vi "Write test data to sql database.vi"(6 "error in (no error)":errorcluster, 9 "Serial":string) -> (0 "error out":errorcluster, 1 "No dup serial?":bool, 2 "Test rec csv line":string, 3 "Passed?":bool)   [LabVIEW 2013]
uses:
  Test Globals/Global 1.vi
  Main Support/Global 2.vi
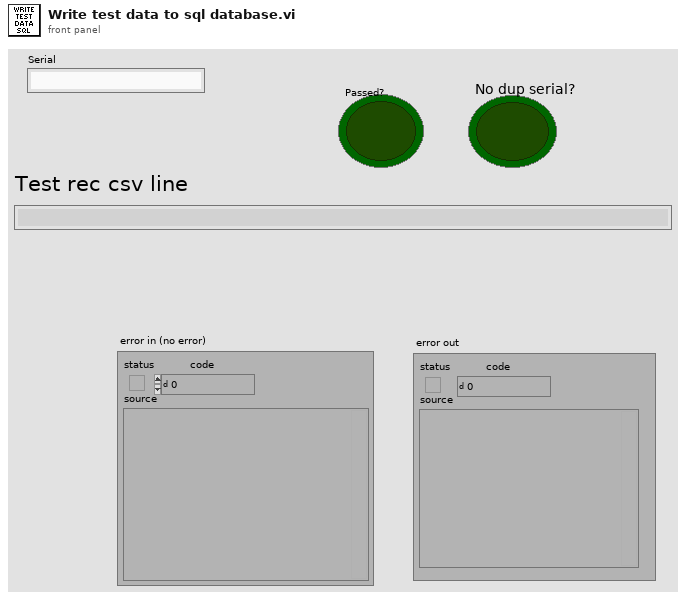
[diagram p1: front panel]
types:
  T1 = enum16{"Query", "Insert", "Select", "Dump Recs", "Get Rec Count", "Get Col Names", "Insert all fields", "Find", "Get last test result", "Get work order qty", "Set work order qty", "Save test report", "Get test report", "Execute query no data", "Select count", "Query and return row 0 col 0"}
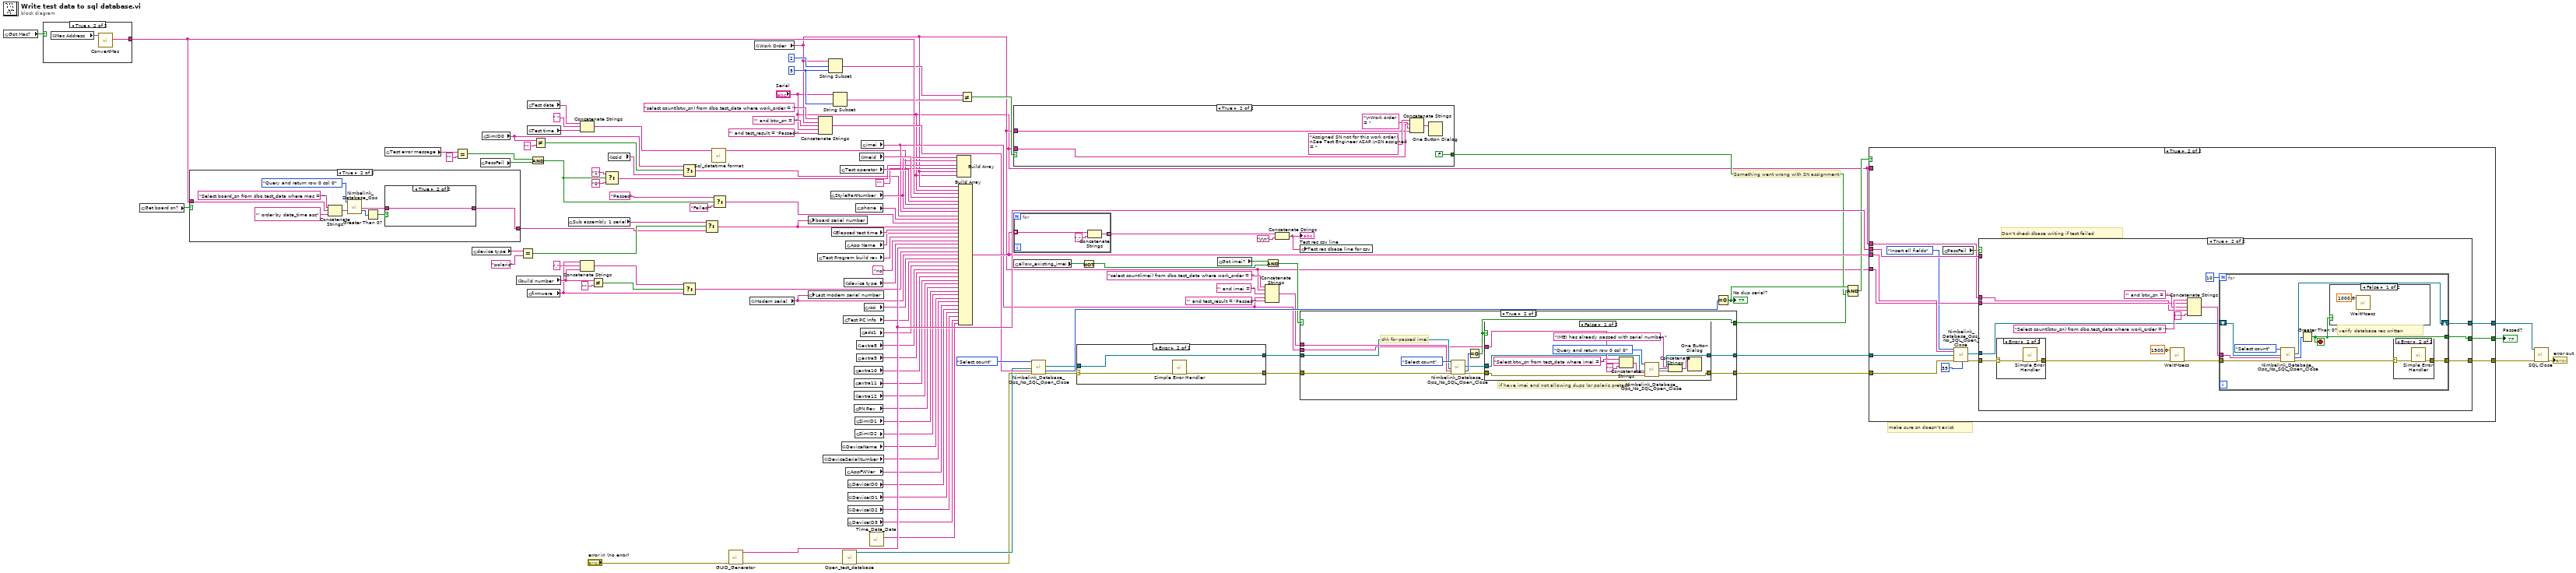
[diagram p0: block diagram]
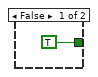
[diagram p2: hidden frame]
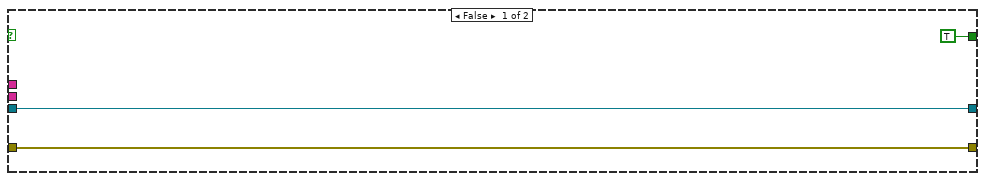
[diagram p3: hidden frame]
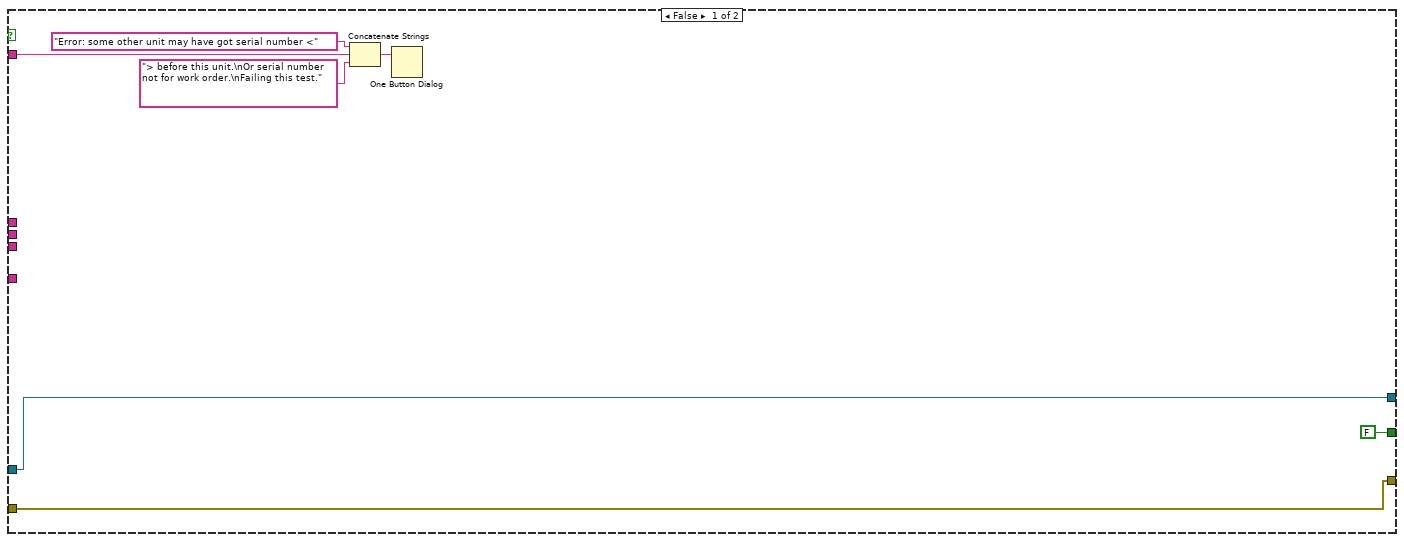
[diagram p6: hidden frame]
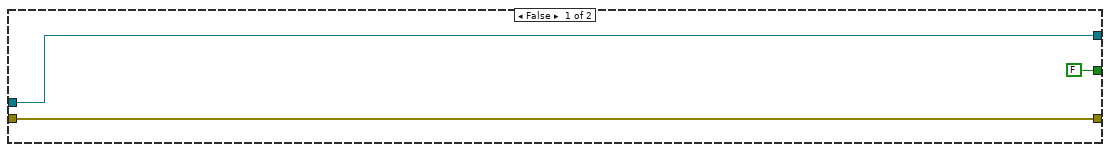
[diagram p7: hidden frame]
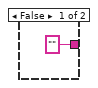
[diagram p11: hidden frame]
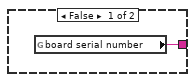
[diagram p12: hidden frame]
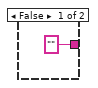
[diagram p13: hidden frame]
diagram:
  w55 = 5 ("length (rest)")
  # "Something went wrong with SN assignment"
  # "make sure sn doesn't exist"
  n1 = global read "Global 1.vi" "Got Mac?"() -> (w93:bool)
  n2 = case shown="True" w93 {
    tunnel: ["" ("Mac without semi") w114] -> w94
    frame False {
    }
    frame True {
      n3 = global read "Global 1.vi" "Mac Address"() -> (w115:string)
      n4 = call "ConvertMac.vi"("Mac (with or without semicolons)"=w115) -> ("Mac without semi"=w114:string)  [unwired: 8 in, 2 out]
    }
  }
  n5 = global read "Global 1.vi" "Get board sn?"() -> (w95:bool)
  n6 = case shown="True" w95 {
    tunnel: [w116 w120] -> w42
    tunnel: w94 -> [_ w119]
    frame False {
      n7 = global read "Global 1.vi" "board serial number"() -> (w116:string)
    }
    frame True {
      n8 = Concatenate Strings("Select board_sn from dbo.test_data where mac = '" ("string"), w119, "' order by date_time asc" ("string")) -> (w123:string)
      n9 = call "Nimbelink_Database_Ops.vi"("Operation"=T1."Query and return row 0 col 0", "SQL Query"=w123) -> ("Find return string"=w117:string, "Records"=w122:i32)  [unwired: 10 in, 6 out]
      n10 = Greater Than 0?(x=w122) -> (x > 0?=w121:bool)
      n11 = case shown="True" w121 {
        tunnel: ["" ("String") w127] -> w120
        tunnel: w117 -> [_ w127]
        frame False {
        }
        frame True {
        }
      }
    }
  }
  n12 = global read "Global 1.vi" "Test error message"() -> (w100:string)
  n13 = Equal?(x=w100, y="") -> (x = y?=w98:bool)
  n14 = global read "Global 1.vi" "device type"() -> (w46:string)
  n15 = global read "Global 2.vi" "PassFail"() -> (w96:bool)
  n16 = global read "Global 1.vi" "SimID0"() -> (w14:string)
  n17 = global read "Global 1.vi" "build number"() -> (w10:string)
  n18 = Equal?(x=w46, y="polaris") -> (x = y?=w44:bool)
  n19 = global read "Global 2.vi" "Test date"() -> (w111:string)
  n20 = global read "Global 2.vi" "Test time"() -> (w109:string)
  n21 = global read "Global 1.vi" "firmware"() -> (w7:string)
  n22 = And(x=w98, y=w96) -> (x .and. y?=w36:bool)
  n23 = Not Equal?(x=w14, y="") -> (x != y?=w15:bool)
  n24 = global read "Global 1.vi" "Sub assembly 1 serial"() -> (w43:string)
  n25 = Concatenate Strings(w111, " " ("string"), w109) -> (w32:string)
  n26 = Concatenate Strings(w7, "." ("string"), w10) -> (w8:string)
  n27 = Not Equal?(x=w10, y="") -> (x != y?=w9:bool)
  n28 = Select(t="1", s=w36, f="0") -> (s? t:f=w31:string)
  n29 = global read "Global 1.vi" "ccid"() -> (w13:string)
  n30 = Select(t=w14, s=w15, f=w13) -> (s? t:f=w26:string)
  n31 = Select(t=w8, s=w9, f=w7) -> (s? t:f=w6:string)
  n32 = Select(t=w43, s=w44, f=w42) -> (s? t:f=w41:string)
  n33 = call "Sql_datetime format.vi"("Date time In"=w32) -> ("Sql datetime type 20"=w29:string)  [unwired: 9 in, 1 out]
  n34 = Select(t="Passed" ("element"), s=w36, f="Failed" ("element")) -> (s? t:f=w101:string)
  n35 = call "GUID_Generator.vi"("error in (no error)"="error in (no error)") -> ("error out"=w89:errorcluster, "GUID String"=w92:string)  [unwired: 9 in]
  n36 = global read "Global 1.vi" "Modem serial"() -> (w58:string)
  n37 = global read "Global 2.vi" "Work Order"() -> (w28:string)
  n38 = global write "Global 1.vi" "board serial number"(w41) -> ()
  n39 = global write "Global 2.vi" "Last modem serial number"(w58) -> ()
  n40 = global read "Global 2.vi" "Test Program build rev"() -> (w103:string)
  n41 = Concatenate Strings("select count(btw_sn) from dbo.test_data where work_order = '" ("SQL Query"), w28, "' and btw_sn = '" ("string"), "Serial", "' and test_result = 'Passed'" ("string")) -> (w74:string)
  n42 = global read "Global 1.vi" "DeviceSerialNumber"() -> (w22:string)
  n43 = String Subset(string=w28, offset (0)=2, length (rest)=w55) -> (substring=w54:string)
  n44 = global read "Global 2.vi" "StylePartNumber"() -> (w33:string)
  n45 = global read "Global 2.vi" "Elapsed test time"() -> (w105:string)
  n46 = String Subset(string="Serial", length (rest)=w55) -> (substring=w53:string)  [unwired: 1 in]
  n47 = global read "Global 2.vi" "Test operator"() -> (w107:string)
  n48 = global read "Global 1.vi" "DeviceName"() -> (w23:string)
  n49 = call "Open_test_database.vi"("error in (no error)"=w89) -> ("error out"=w2:errorcluster, "SQL conn Refnum out"=w72:refnum<k7>)  [unwired: 9 in]
  n50 = global read "Global 2.vi" "Test PC Info"() -> (w85:string)
  n51 = global read "Global 1.vi" "device type"() -> (w91:string)
  n52 = global read "Global 2.vi" "App Name"() -> (w104:string)
  n53 = global read "Global 1.vi" "AppFWVer"() -> (w21:string)
  n54 = global read "Global 1.vi" "DeviceID0"() -> (w20:string)
  n55 = global read "Global 1.vi" "DeviceID1"() -> (w19:string)
  n56 = global read "Global 1.vi" "DeviceID2"() -> (w18:string)
  n57 = global read "Global 1.vi" "DeviceID3"() -> (w17:string)
  n58 = global read "Global 1.vi" "extra10"() -> (w62:string)
  n59 = global read "Global 1.vi" "extra11"() -> (w61:string)
  n60 = global read "Global 1.vi" "extra12"() -> (w60:string)
  n61 = global read "Global 2.vi" "PN Rev"() -> (w37:string)
  n62 = global read "Global 1.vi" "SimID1"() -> (w25:string)
  n63 = global read "Global 1.vi" "SimID2"() -> (w24:string)
  n64 = global read "Global 1.vi" "phone"() -> (w106:string)
  n65 = global read "Global 1.vi" "extra8"() -> (w64:string)
  n66 = global read "Global 1.vi" "extra9"() -> (w63:string)
  n67 = global read "Global 1.vi" "meid"() -> (w108:string)
  n68 = global read "Global 1.vi" "adc1"() -> (w83:string)
  n69 = global read "Global 1.vi" "imei"() -> (w57:string)
  n70 = global read "Global 1.vi" "rssi"() -> (w86:string)
  n71 = call "Time_Date_Data.vi"() -> ("UTC ISO 8601"=w5:string)  [unwired: 4 in, 7 out]
  n72 = Build Array(w33, w29, w31, "", w28, "Serial") -> ()  [unwired: 1 out]
  n73 = Build Array(w28, "Serial", w94, w108, w107, w29, w33, w57, w26, w106, w101, w41, w105, w104, w103, "no" ("element"), w91, w92, w6, w58, w86, w85, w83, w64, w63, w62, w61, w60, w37, w25, w24, w23, w22, w21, w20, w19, w18, w17, w5) -> (w82:string[])
  n74 = Not Equal?(x=w54, y=w53) -> (x != y?=w52:bool)
  n75 = case shown="True" w52 {
    tunnel: "Serial" -> [_ w132]
    tunnel: w28 -> [_ w130]
    tunnel: [TRUE FALSE] -> w49
    frame False {
    }
    frame True {
      n76 = Concatenate Strings("Assigned SN not for this work order.\nSee Test Engineer ASAP.\nSN assigned = " ("string"), w132, "\nWork order = " ("string"), w130) -> (w134:string)
      n77 = One Button Dialog(message=w134) -> ()  [unwired: 1 in, 1 out]
    }
  }
  n78 = for {
    tunnel: w82 -> [w137] mode=indexing
    tunnel: [w135] -> w81 mode=indexing
    n79 = Concatenate Strings(w137, "," ("string")) -> (w135:string)
  }
  n80 = global read "Global 1.vi" "allow_existing_imei"() -> (w39:bool)
  n81 = call "Nimbelink_Database_Ops_No_SQL_Open_Close.vi"("Operation"=T1."Select count", "Connection In"=w72, "SQL Query"=w74, "Error in (no error)"=w2) -> ("Connection Out"=w66:refnum<k7>, "Records"=w73:i32, "Error out"=w1:errorcluster)  [unwired: 8 in, 5 out]
  n82 = case shown="Error" w1 {
    selector: w1 -> [w139 w142]
    tunnel: [w139 w141] -> w67
    tunnel: w66 -> [w138 w140]
    tunnel: [w138 w140] -> w65
    frame No Error {
    }
    frame Error {
      n83 = call <vilib>:"Simple Error Handler.vi"("error in (no error)"=w142) -> ("error out"=w141:errorcluster)  [unwired: 4 in, 4 out]
    }
  }
  n84 = Not(x=w39) -> (.not. x?=w40:bool)
  n85 = global read "Global 1.vi" "Got imei?"() -> (w59:bool)
  n86 = Concatenate Strings("select count(imei) from dbo.test_data where work_order = '" ("SQL Query"), w28, "' and imei = '" ("string"), w57, "' and test_result = 'Passed'" ("string")) -> (w68:string)
  n87 = And(x=w59, y=w40) -> (x .and. y?=w38:bool)
  n88 = Concatenate Strings(w81, "\r\n") -> (w79:string)
  "Test rec csv line" <- w79
  n89 = global write "Global 1.vi" "Test rec dbase line for csv"(w79) -> ()
  n90 = case shown="True" w38 {
    tunnel: w68 -> [_ w155]
    tunnel: [TRUE w151] -> w50
    tunnel: w67 -> [w144 w153]
    tunnel: [w144 w150] -> w3
    tunnel: w65 -> [w143 w152]
    tunnel: [w143 w147] -> w4
    tunnel: w57 -> [_ w149]
    frame False {
    }
    frame True {
      # "if have imei and not allowing dups (or polaris pretest)"
      # "chk for passed imei"
      n91 = call "Nimbelink_Database_Ops_No_SQL_Open_Close.vi"("Operation"=T1."Select count", "Connection In"=w152, "SQL Query"=w155, "Error in (no error)"=w153) -> ("Connection Out"=w148:refnum<k7>, "Records"=w154:i32, "Error out"=w146:errorcluster)  [unwired: 8 in, 5 out]
      n92 = Equal To 0?(x=w154) -> (x = 0?=w151:bool)
      n93 = case shown="False" w151 {
        tunnel: w146 -> [w168 w170]
        tunnel: [w167 w170] -> w150
        tunnel: w149 -> [w164 _]
        tunnel: w148 -> [w158 w169]
        tunnel: [w157 w169] -> w147
        frame False {
          n94 = Concatenate Strings("Select btw_sn from test_data where imei = '" ("SQL Query"), w164, "'" ("string")) -> (w162:string)
          n95 = call "Nimbelink_Database_Ops_No_SQL_Open_Close.vi"("Operation"=T1."Query and return row 0 col 0", "Connection In"=w158, "SQL Query"=w162, "Error in (no error)"=w168) -> ("Connection Out"=w157:refnum<k7>, "Find return string"=w160:string, "Error out"=w167:errorcluster)  [unwired: 8 in, 5 out]
          n96 = Concatenate Strings("IMEI has already passed with serial number " ("message"), w160) -> (w159:string)
          n97 = One Button Dialog(message=w159) -> ()  [unwired: 1 in, 1 out]
        }
        frame True {
        }
      }
    }
  }
  n98 = Equal To 0?(x=w73) -> (x = 0?=w51:bool)
  "No dup serial?" <- w51
  n99 = Compound Arithmetic op=AND(w51, w50, w49) -> (w48:bool)
  n100 = case shown="True" w48 {
    tunnel: [FALSE w191] -> w47
    tunnel: w92 -> [_ w190]
    tunnel: w4 -> [w176 w189]
    tunnel: [w177 w188] -> w88
    tunnel: [w176 w187] -> w87
    tunnel: w82 -> [_ w186]
    tunnel: w28 -> [_ w185]
    tunnel: "Serial" -> [_ w184]
    tunnel: w3 -> [w177 w183]
    tunnel: "Serial" -> [w173 _]
    frame False {
      n101 = Concatenate Strings("Error: some other unit may have got serial number <" ("message"), w173, "> before this unit.\nOr serial number not for work order.\nFailing this test." ("string")) -> (w171:string)
      n102 = One Button Dialog(message=w171) -> ()  [unwired: 1 in, 1 out]
    }
    frame True {
      # "Don't check dbase writing if test failed"
      n103 = global read "Global 2.vi" "PassFail"() -> (w180:bool)
      n104 = call "Nimbelink_Database_Ops_No_SQL_Open_Close.vi"("Operation"=T1."Insert all fields", "Record data"=w186, "Connection In"=w189, "Error in (no error)"=w183, "Insert fields"=39) -> ("Connection Out"=w181:refnum<k7>, "Error out"=w178:errorcluster)  [unwired: 7 in, 6 out]
      n105 = case shown="True" w180 {
        tunnel: w190 -> [_ _]
        tunnel: [FALSE w206] -> w191
        tunnel: [w194 w205] -> w188
        tunnel: w178 -> [w194 w197]
        tunnel: w181 -> [w193 w201]
        tunnel: [w193 w195] -> w187
        tunnel: w185 -> [_ w200]
        tunnel: w184 -> [_ w199]
        frame False {
        }
        frame True {
          n106 = case shown="Error" w197 {
            selector: w197 -> [w210 w212]
            tunnel: [w210 w211] -> w196
            frame No Error {
            }
            frame Error {
              n107 = call <vilib>:"Simple Error Handler.vi"("error in (no error)"=w212) -> ("error out"=w211:errorcluster)  [unwired: 4 in, 4 out]
            }
          }
          n108 = call "WaitMsecs.vi"("error in (no error)"=w196, "Wait Msecs"=1500.0) -> ("error out"=w202:errorcluster)  [unwired: 9 in]
          n109 = Concatenate Strings("Select count(btw_sn) from dbo.test_data where work_order = '" ("SQL Query"), w200, "' and btw_sn = '" ("string"), w199, "'" ("string")) -> (w207:string)
          n110 = for {
            N: 10 -> [_]
            tunnel: w207 -> [w221]
            tunnel: [w220] -> w206
            tunnel: [w215] -> w205
            tunnel: w202 -> [w219]
            shift-right: [w214] -> w195
            shift-left: w201 -> [w216]
            stop <- w220 stop-if-true
            # "verify database rec written"
            n111 = call "Nimbelink_Database_Ops_No_SQL_Open_Close.vi"("Operation"=T1."Select count", "Connection In"=w216, "SQL Query"=w221, "Error in (no error)"=w219) -> ("Connection Out"=w214:refnum<k7>, "Records"=w217:i32, "Error out"=w213:errorcluster)  [unwired: 8 in, 5 out]
            n112 = Greater Than 0?(x=w217) -> (x > 0?=w220:bool)
            n113 = case shown="False" w220 {
              frame False {
                n114 = call "WaitMsecs.vi"("Wait Msecs"=1000.0) -> ()  [unwired: 10 in, 1 out]
              }
              frame True {
              }
            }
            n115 = case shown="Error" w213 {
              selector: w213 -> [w222 w224]
              tunnel: [w222 w223] -> w215
              frame No Error {
              }
              frame Error {
                n116 = call <vilib>:"Simple Error Handler.vi"("error in (no error)"=w224) -> ("error out"=w223:errorcluster)  [unwired: 4 in, 4 out]
              }
            }
          }
        }
      }
    }
  }
  "Passed?" <- w47
  n117 = call "SQL Close.vi"("Connection In"=w87, "Error in (no error)"=w88) -> ("Error out"=→"error out":errorcluster)  [unwired: 17 in]
